vi "checkPython2.vi"(8 "error in (no error)":errorcluster) -> (0 "error out":errorcluster)   [LabVIEW 2016]
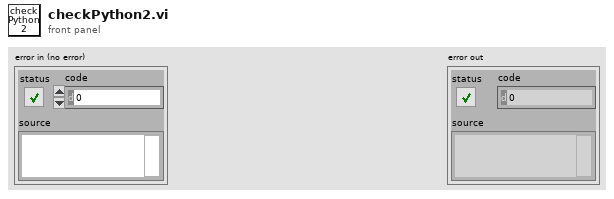
[diagram p1: front panel]
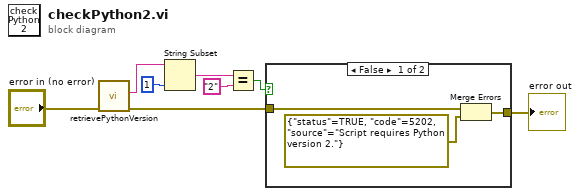
[diagram p0: block diagram]
diagram:
  n1 = call "retrievePythonVersion.vi"("error in (no error)"="error in (no error)") -> ("error out"=w2:errorcluster, "Python version"=w8:string)  [unwired: 9 in]
  n2 = String Subset(string=w8, length (rest)=1 ("length (rest)")) -> (substring=w6:string)  [unwired: 1 in]
  n3 = Equal?(x=w6, y="2") -> (x = y?=w4:bool)
  n4 = case shown="False" w4 {
    tunnel: w2 -> [w11 w12]
    tunnel: [w9 w12] -> w1
    frame False {
      n5 = Merge Errors(w11, errorcluster {"status"=TRUE, "code"=5202, "source"="Script requires Python version 2."} ("error constant")) -> (w9:errorcluster)
    }
    frame True {
    }
  }
  "error out" <- w1
